vi "TB-Adjust Level.vi"(0 "Stimulus In":T22(xcontrol), 7 "Meas SPL":dbl, 9 "Max SPL History":dbl[](array[numeric]), 11 "error in (no error)":errorcluster, 12 "Tolerance (dB)":dbl=0.5, 13 "Adjust?":bool) -> (4 "Stimulus Out":T22(xcontrol), 8 "Meas SPL out":dbl, 10 "Max SPL History out":dbl[](array[numeric]), 14 "Max SPL":dbl, 15 "error out":errorcluster)   [LabVIEW 2020]
uses:
  epl-vi-lib/Signal Synthesis VIs/Controls/Stimulus Channel XCtl/Stimulus Channel.xctl
  <vilib>/Analysis/baseanly.llb/Mean (DBL).vi
  <vilib>/Analysis/NI_AALBase.lvlib
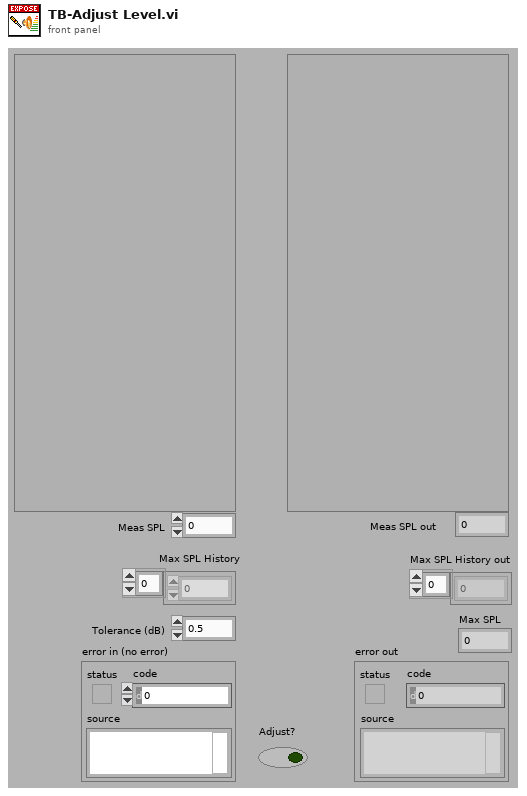
[diagram p1: front panel]
types:
  T1 = typedef "Waveform XCtl.xctl/Waveform Data.ctl" = cluster{"Type":T2, "Tone":T3, "Pulse Train":T4, "Noise":T7, "File":T8, "FMSweep":T9, "Chirp Train":T10, "Complex Tone":cluster{"Params":T12, "Data":T14}, "Moving Ripple":T15}
  T2 = typedef "Waveform Enum.ctl" = enum16{"OFF", "Tone", "Noise", "Pulse Train", "File", "FM Sweep", "Chirp Train", "Complex Tone", "FM Tone", "Moving Ripple"}
  T3 = typedef "Tone Params.ctl" = cluster{"Frequency (kHz)":dbl, "Last Freq":dbl, "Last Phase":dbl}
  T4 = typedef "Pulse Train Params.ctl" = cluster{"Pulse width (us)":dbl, "Pulse rate (Hz)":dbl, "Gap (ms)":dbl, "Polarity":T5, "PT State":T6, "Asynch":bool}
  T5 = typedef "Pulse Polarity.ctl" = enum16{"POS", "NEG", "POS-NEG", "NEG-POS"}
  T6 = typedef "PT-Continuous State.ctl" = cluster{"Template":dbl[], "Nperiod":i32, "Index":i32, "Pulse Rate (Hz)":dbl, "Phase (cycles)":dbl, "Noff":i32}
  T7 = typedef "Noise Params.ctl" = cluster{"InvFilt":bool, "Noise":dbl[], "CurPt":i32, "Aweight":bool, "Seed":i32, "afile":path}
  T8 = typedef "StimFile-Params.ctl" = cluster{"Filename":path, "Signal":dbl[], "Channel":i32, "stream":bool, "offset":i32, "nreps":i32, "loops":i32, "Randomize":bool, "order":i32[], "Seed":i32, "Tokens":i32}
  T9 = typedef "FM Sweep Params.ctl" = cluster{"Rate (oct/s)":dbl, "Fmin (Hz)":dbl, "Fmax (Hz)":dbl, "Ramp (ms)":dbl, "Linear":bool}
  T10 = typedef "Chirp Train.ctl" = cluster{"Params":T11, "Data":cluster{"WF":dbl[]}}
  T11 = typedef "Chirp Train Params.ctl" = cluster{"Fmin (kHz)":dbl, "Fmax (kHz)":dbl, "Compensate":bool, "Duration (ms)":dbl}
  T12 = typedef "CT-Params.ctl" = cluster{"F0 (Hz)":dbl, "Band":cluster{"Flow (Hz)":dbl, "Fhigh (Hz)":dbl}, "Phase":T13, "Min F0 (Hz)":dbl, "Max F0 (Hz)":dbl, "ContinRandPhase":bool, "Max peak factor":dbl, "Max mod depth":dbl, "MinHarmNum":i32, "MaxHarmNum":i32, "Level Mode":enum16{"per component", "overall rms"}, "% jitter":dbl}
  T13 = typedef "CT-Phase Enum.ctl" = enum16{"Cosine", "Random", "Alternating"}
  T14 = typedef "CT-Runtime Data.ctl" = cluster{"Ncomp":i32, "MinHarm":i32, "Phase":dbl[], "Amplitude":dbl[], "Npts/frame":i32, "Last F0":dbl, "Fmin":dbl, "Fmax":dbl, "Lslope":dbl, "randphase":bool, "overall rms":bool, "fmult":dbl[], "jittered":bool}
  T15 = typedef "Moving Ripple.ctl" = cluster{"Params":T16, "Data":T17}
  T16 = typedef "Moving Ripple.Params.ctl" = cluster{"Fmin":dbl, "Fmax":dbl, "Density":dbl, "Velocity":dbl, "Depth":dbl, "Phase":dbl, "Comp/oct":i32}
  T17 = typedef "Moving Ripple.Data.ctl" = cluster{"Freq":dbl[], "A":dbl[], "phase":dbl[], "Phase":dbl}
  T18 = typedef "Filter XCtl.xctl/Filter Data.ctl" = cluster{"CF (kHz)":dbl, "BW (kHz)":dbl, "IIR Filter Cluster":cluster{"filter structure":enum32{"IIR 2nd Order", "IIR 4th Order"}, "Reverse Coefficients":dbl[], "Forward Coefficients":dbl[]}, "Final Filter State":dbl[], "Scale Factor":dbl, "Final Filter State 2":dbl[], "Quadrature":bool, "Type":enum16{"Lowpass", "Highpass", "Bandpass", "Bandstop", "OFF"}}
  T19 = typedef "Gate Control.xctl/Gate Data.ctl" = cluster{"Active":bool, "Delay (ms)":dbl, "Width (ms)":dbl, "Ramp (ms)":dbl}
  T20 = typedef "Level XCtl.xctl/Level Data.ctl" = cluster{"Level":dbl, "Units":T21, "Max":dbl, "Multiplier":dbl, "Cal File":path, "Cal":cluster{"Freq (Hz)":dbl[], "Mag (dB SPL)":dbl[], "Phase (deg)":dbl[]}}
  T21 = typedef "Level Units.ctl" = enum16{"dB atten", "dB SPL", "dB re 1 Vrms", "dB V/Hz½", "mW", "dB HL", "Volts", "dB mW"}
  T22 = cluster{"Waveform":T1, "Filter":T18, "Gate":T19, "Level":T20}
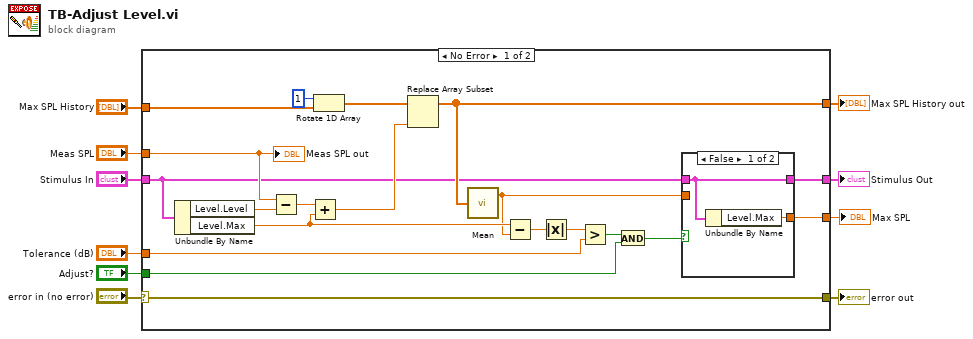
[diagram p0: block diagram]
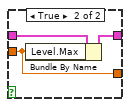
[diagram p2: hidden frame]
diagram:
  n1 = case shown="No Error" "error in (no error)" {
    selector: "error in (no error)" -> [w12 w36]
    tunnel: "Max SPL History" -> [w28 _]
    tunnel: "Meas SPL" -> [w23 _]
    tunnel: [w22 _] -> w8
    tunnel: "Tolerance (dB)" -> [w19 _]
    tunnel: "Adjust?" -> [w17 _]
    tunnel: "Stimulus In" -> [w14 _]
    tunnel: [w13 _] -> w4
    tunnel: [w12 w36] -> w2
    tunnel: [w11 _] -> w1
    frame No Error {
      n2 = Unbundle By Name(w14) -> ("Level.Level"=w30:dbl, "Level.Max"=w24:dbl)
      n3 = Subtract(x=w23, y=w30) -> (x-y=w29:dbl)
      n4 = Add(x=w29, y=w24) -> (x+y=w25:dbl)
      n5 = Rotate 1D Array(1:w28, 2:1 ("n")) -> (0:w26:dbl[])
      n6 = Replace Array Subset(array=w26, new element=w25) -> (w22:dbl[])  [unwired: 1 in]
      n7 = call-poly <vilib>:"Mean.vi"("X"=w22) -> ("mean"=w16:dbl)  [unwired: 1 out]
      n8 = Subtract(x=w24, y=w16) -> (x-y=w21:dbl)
      n9 = Absolute Value(x=w21) -> (abs(x)=w20:dbl)
      n10 = Greater?(x=w20, y=w19) -> (0:w18:bool)
      n11 = And(x=w18, y=w17) -> (x .and. y?=w15:bool)
      n12 = case shown="False" w15 {
        tunnel: w16 -> [_ w33]
        tunnel: w14 -> [w32 w35]
        tunnel: [w32 w34] -> w13
        tunnel: [w31 w33] -> w11
        frame False {
          n13 = Unbundle By Name(w32) -> ("Level.Max"=w31:dbl)
        }
        frame True {
          n14 = Bundle By Name(cluster=w35, "Level.Max"=w33) -> (w34:T22)
        }
      }
      "Meas SPL out" <- w23
    }
    frame Error {
    }
  }
  "error out" <- w2
  "Stimulus Out" <- w4
  "Max SPL History out" <- w8
  "Max SPL" <- w1
